vi "Generate Report Set Modified Data.vi"(4 "error in (no error)":errorcluster, 6 "data":T1, 7 "report in":T2) -> (0 "error out":errorcluster, 3 "report out":T2)   [LabVIEW 2012, in "NISH Report.lvlib"]
doc: "This VI overwrites the data associated with the <B>Generate Report</B> object reference and unlocks it for write access. If <B>error in</B> is set, the object is unlocked but its data will not be modified.\n\nIn order to use this VI, you must first successfully lock the object's data using the <B>Generate Report Get Data To Modify</B> VI.\n\n[GOOP 1.0/1.0]"
uses:
  <resource>/importtools/NISH Report/NISH Report.lvlib
  <resource>/importtools/NISH Report/Generate Report Data Members.ctl
  <resource>/importtools/NISH Report/Generate Report Object Reference.ctl
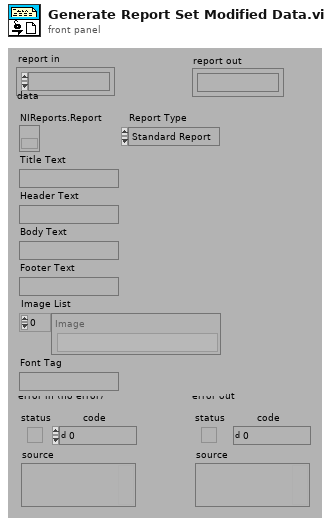
[diagram p1: front panel]
types:
  T1 = typedef "NISH Report.lvlib/Generate Report Data Members.ctl" = cluster{"Title Text":string, "Header Text":string, "Body Text":string, "Footer Text":string, "Image List":string[], "NIReports.Report":refnum<k7>, "Report Type":enum16{"Standard Report", "HTML"}, "Font Tag":string}
  T2 = typedef "NISH Report.lvlib/Generate Report Object Reference.ctl" = refnum<k1>
  T3 = enum16{"Create", "GetCopy", "GetModify", "Set", "Destroy", "Create Static", "Get All Refs", "Reset", "Get Statistics"}
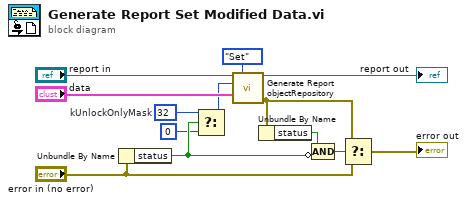
[diagram p0: block diagram]
diagram:
  w3 = 32  # kUnlockOnlyMask
  n1 = Unbundle By Name("error in (no error)") -> ("status"=w4:bool)
  n2 = Select(t=w3, s=w4, f=0 ("flags in")) -> (s? t:f=w1:i32)
  n3 = call <resource>:"Generate Report objectRepository.vi"("reference in"="report in", "method"=T3."Set", "flags in"=w1, "classDataIn"="data") -> ("reference out"=→"report out":T2, "error out"=w8:errorcluster)  [unwired: 5 in, 5 out]
  n4 = Unbundle By Name(w8) -> ("status"=w9:bool)
  n5 = Compound Arithmetic op=AND(w9, invert w4) -> (w10:bool)
  n6 = Select(t=w8, s=w10, f="error in (no error)") -> (s? t:f=→"error out":errorcluster)
